vi "Get Rx UDP All Channels.vi"(8 "error in":errorcluster, 11 "custom device ref in":T1 format="%.0x") -> (0 "error out":errorcluster, 2 "Rx UDP channel refs":T1[](array[typedef]) format="%.0x", 3 "custom device ref out":T1 format="%.0x")   [LabVIEW 2020, in "AIM ARINC 664 Scripting.lvlib"]
uses:
  AIM ARINC 664 Scripting.lvlib
  <vilib>/NI VeriStand/Custom Device Tools/Custom Device Utility Library/Custom Device Utility Library.lvlib
  Constants.vi
  <vilib>/NI VeriStand/Custom Device API/Custom Device API.lvlib
  <vilib>/NI VeriStand/Custom Device Tools/Custom Device Utility Library/NI VeriStand - Search for All Items by GUID.vi
  <vilib>/NI VeriStand/Custom Device Tools/Custom Device Utility Library/NI VeriStand - Search for Item by GUID.vi
  <vilib>/NI VeriStand/Custom Device API/Custom Device Item Ref.ctl
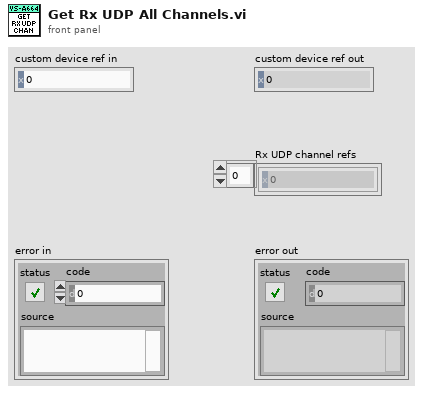
[diagram p1: front panel]
types:
  T1 = typedef "Custom Device API.lvlib/Custom Device Item Ref.ctl" = u64
  T2 = typedef "Custom Device API.lvlib/Custom Device Item Info.ctl" = cluster{"Name":string, "Is Channel":bool, "GUID":string, "Is Waveform":bool}
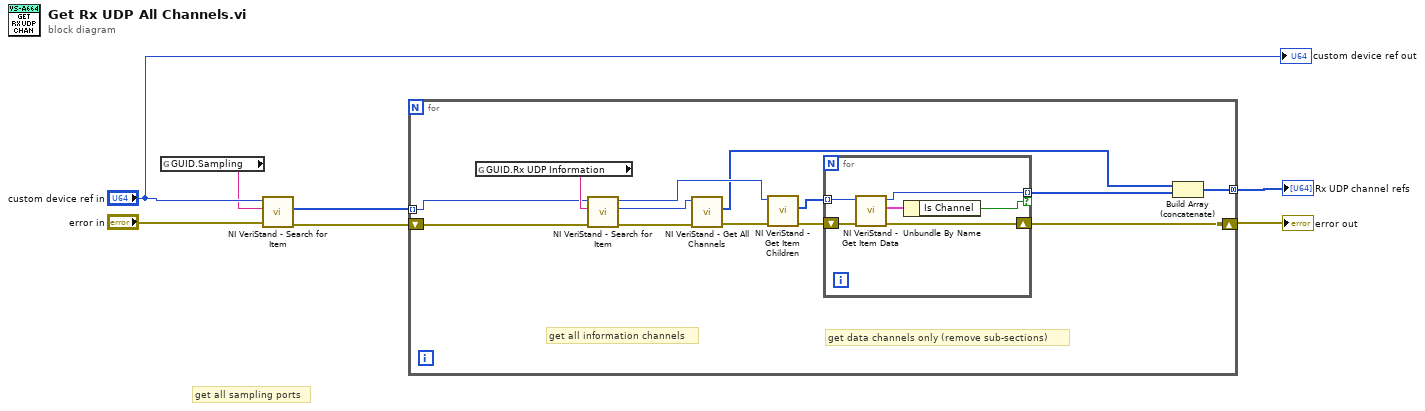
[diagram p0: block diagram]
diagram:
  # "get all sampling ports"
  n1 = global read "Constants.vi" "GUID.Sampling"() -> (w3:string)
  n2 = call-poly <vilib>:"NI VeriStand - Search for Item.vi"("error in"="error in", "Item GUID"=w3, "Section Ref in"="custom device ref in") -> ("error out"=w1:errorcluster, "Item Refs"=w2:T1[])  [unwired: 5 in, 2 out]
  n3 = for {
    tunnel: w2 -> [w10] mode=indexing
    shift-right: [w11] -> w7
    shift-left: w1 -> [w20]
    tunnel: [w13] -> w6 mode=concatenating
    # "get data channels only (remove sub-sections)"
    # "get all information channels"
    n4 = global read "Constants.vi" "GUID.Rx UDP Information"() -> (w19:string)
    n5 = call-poly <vilib>:"NI VeriStand - Search for Item.vi"("error in"=w20, "Item GUID"=w19, "Section Ref in"=w10) -> ("error out"=w18:errorcluster, "Item Ref"=w17:T1, "Section Ref out"=w12:T1)  [unwired: 5 in, 1 out]
    n6 = call <vilib>:"NI VeriStand - Get All Channels.vi"("error in"=w18, "Section Ref in"=w17) -> ("error out"=w16:errorcluster, "Channel Refs"=w9:T1[])  [unwired: 6 in, 2 out]
    n7 = call <vilib>:"NI VeriStand - Get Item Children.vi"("error in (no error)"=w16, "Item Ref in"=w12) -> ("error out"=w15:errorcluster, "Child Refs"=w14:T1[])  [unwired: 6 in, 2 out]
    n8 = for {
      shift-right: [w21] -> w11
      shift-left: w15 -> [w22]
      tunnel: w14 -> [w26] mode=indexing
      tunnel: [w24] -> w8 mode=indexing if=w23
      n9 = call <vilib>:"NI VeriStand - Get Item Data.vi"("error in (no error)"=w22, "Item Ref in"=w26) -> ("error out"=w21:errorcluster, "Item Info"=w25:T2, "Item Ref out"=w24:T1)  [unwired: 7 out]
      n10 = Unbundle By Name(w25) -> ("Is Channel"=w23:bool)
    }
    n11 = Build Array (concatenate)(w9, w8) -> (w13:T1[])
  }
  "error out" <- w7
  "Rx UDP channel refs" <- w6
  "custom device ref out" <- "custom device ref in"
